vi "Stop XRT-U.vi"(8 "error in (no error)":errorcluster, 11 "Inst.Xeryon-Rotator in":refnum<class "Inst.Xeryon-Rotator.lvclass">) -> (0 "error out":errorcluster, 3 "Inst.Xeryon-Rotator out":refnum<class "Inst.Xeryon-Rotator.lvclass">)   [LabVIEW 2019, in "Inst.Xeryon-Rotator.lvclass"]
uses:
  Inst.Xeryon-Rotator.lvclass
  Inst.Xeryon-Rotator.lvclass/Inst.Xeryon-Rotator.ctl
  drivers/Class/Controller/Controller.lvclass
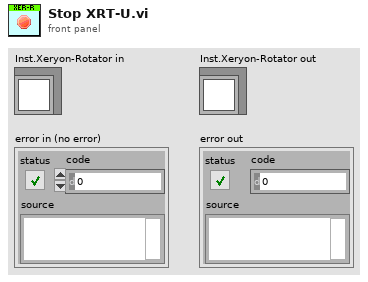
[diagram p1: front panel]
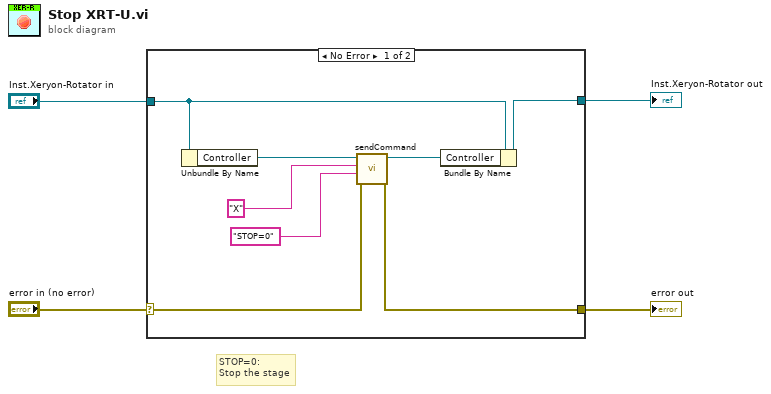
[diagram p0: block diagram]
diagram:
  # "STOP=0:\nStop the stage"
  n1 = case shown="No Error" "error in (no error)" {
    selector: "error in (no error)" -> [w5 w14]
    tunnel: [w12 w13] -> w1
    tunnel: [w7 w14] -> w2
    tunnel: "Inst.Xeryon-Rotator in" -> [w6 w13]
    frame No Error {
      n2 = Unbundle By Name(w6) -> ("Controller"=w10:refnum<class "Controller.lvclass">)
      n3 = call-dynamic "sendCommand.vi"("error in (no error)"=w5, "Command"="STOP=0", "Axis Letter"="X", "Controller in"=w10) -> ("error out"=w7:errorcluster, "Controller out"=w8:refnum<class "Controller.lvclass">)  [unwired: 6 in]
      n4 = Bundle By Name(cluster=w6, "Controller"=w8) -> (w12:refnum<class "Inst.Xeryon-Rotator.lvclass">)
    }
    frame Error {
    }
  }
  "error out" <- w2
  "Inst.Xeryon-Rotator out" <- w1
